vi "Init.vi"(8 "error in (no error)":errorcluster, 11 "Data in":refnum<class "Local Vars.lvclass">) -> (0 "error out":errorcluster, 3 "Data out":refnum<class "Local Vars.lvclass">)   [LabVIEW 2021, in "Local Vars.lvclass"]
uses:
  Local Vars.lvclass
  Local Vars.lvclass/Local Vars.ctl
  Var Access/Var_Access.lvclass
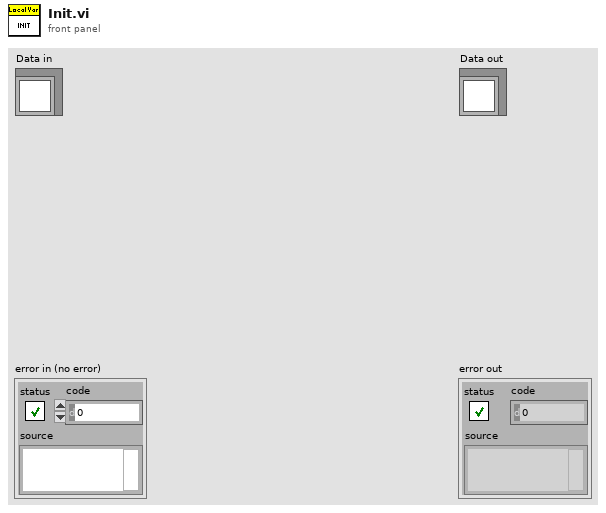
[diagram p1: front panel]
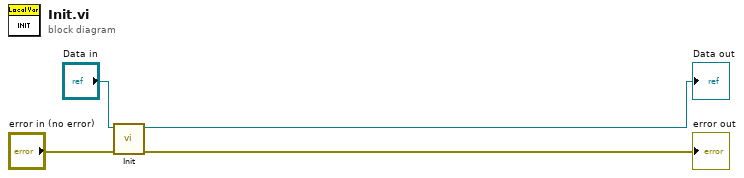
[diagram p0: block diagram]
diagram:
  n1 = call-parent "Init.vi"("error in (no error)"="error in (no error)", "Data in"="Data in") -> ("error out"=→"error out":errorcluster, "Data out"=→"Data out":refnum<class "Local Vars.lvclass">)  [unwired: 8 in]
